vi "Register Tool Buttons Pressed.vi"(8 "error in (no error)":errorcluster, 11 "UI Controller in":refnum<class "UI Controller.lvclass">) -> (0 "error out":errorcluster, 3 "UI Controller out":refnum<class "UI Controller.lvclass">)   [LabVIEW 2020, in "UI Controller.lvlib" / "UI Controller.lvclass"]
uses:
  UI Controller.lvclass
  C:/Program Files/National Instruments/LabVIEW 2020/vi.lib/ActorFrameworkMVC/Abstract Controller/Abstract Controller/Abstract Controller.lvclass
  C:/Program Files/National Instruments/LabVIEW 2020/vi.lib/ActorFramework/Actor/Actor.lvclass
  Views/Tools View/Tools View Messages/Register Tool Buttons Pressed Msg/Register Tool Buttons Pressed Msg.lvclass
  C:/Program Files/National Instruments/LabVIEW 2020/vi.lib/ActorFramework/Message/Message.lvclass
  Models/Map Model/Map Model Messages/Concrete Tool Buttons Pressed Msg/Concrete Tool Buttons Pressed Msg.lvclass
  C:/Program Files/National Instruments/LabVIEW 2020/vi.lib/ActorFrameworkObserver/Data Message/Data Message.lvclass
  <vilib>/ActorFramework/Message Enqueuer/Message Enqueuer.lvclass/Message Enqueuer.ctl
  Views/Map View/Map View Messages/Concrete Tool Buttons Pressed Msg/Concrete Tool Buttons Pressed Msg.lvclass
  UI Controller Messages/Concrete Tool Buttons Pressed Msg/Concrete Tool Buttons Pressed Msg.lvclass
  <vilib>/ActorFramework/Actor/Actor.lvclass/Actor.ctl
  <vilib>/ActorFramework/Message Enqueuer/Init from Existing Queue.vi
  <vilib>/ActorFramework/Message Priority Queue/Priority Enqueue.vi
  <vilib>/ActorFramework/Message Enqueuer/Message Enqueuer.lvclass
  <vilib>/ActorFrameworkMVC/Abstract Controller/Abstract Controller/Abstract Controller.lvclass
  <vilib>/ActorFramework/Actor/Actor.lvclass
panel:
  # "NOTICE -- YOU MUST LEAVE THIS NOTICE IN PLACE.\n\nCopyright (c) 2017, LIANG LIU Shawn.Liu.cn@gmail.com\nAll rights reserved.\n\nRedistribution and use in source and binary forms, with or without modification, are permitted provided that the following conditions are met:\n-Redistributions of source code must retain the above copyright notice, this list of conditions and the following disclaimer.\n-Redistributions in binary form must reproduce the above copyright notice, this list of conditions and the following disclaimer in the documentation and/or other materials provided with the distribution.\n-Neither the name of the eLp nor the names of its contributors may be used to endorse or promote products derived from this software without specific prior written permission.\n\nTHIS SOFTWARE IS PROVIDED BY THE COPYRIGHT HOLDERS AND CONTRIBUTORS \"AS IS\" AND ANY EXPRESS OR IMPLIED WARRANTIES, INCLUDING, BUT NOT LIMITED TO, THE IMPLIED WARRANTIES OF MERCHANTABILITY AND FITNESS FOR A PARTICULAR PURPOSE ARE DISCLAIMED. IN NO EVENT SHALL THE COPYRIGHT HOLDER OR CONTRIBUTORS BE LIABLE FOR ANY DIRECT, INDIRECT, INCIDENTAL, SPECIAL, EXEMPLARY, OR CONSEQUENTIAL DAMAGES (INCLUDING, BUT NOT LIMITED TO, PROCUREMENT OF SUBSTITUTE GOODS OR SERVICES; LOSS OF USE, DATA, OR PROFITS; OR BUSINESS INTERRUPTION) HOWEVER CAUSED AND ON ANY THEORY OF LIABILITY, WHETHER IN CONTRACT, STRICT LIABILITY, OR TORT (INCLUDING NEGLIGENCE OR OTHERWISE) ARISING IN ANY WAY OUT OF THE USE OF THIS SOFTWARE, EVEN IF ADVISED OF THE POSSIBILITY OF SUCH DAMAGE."
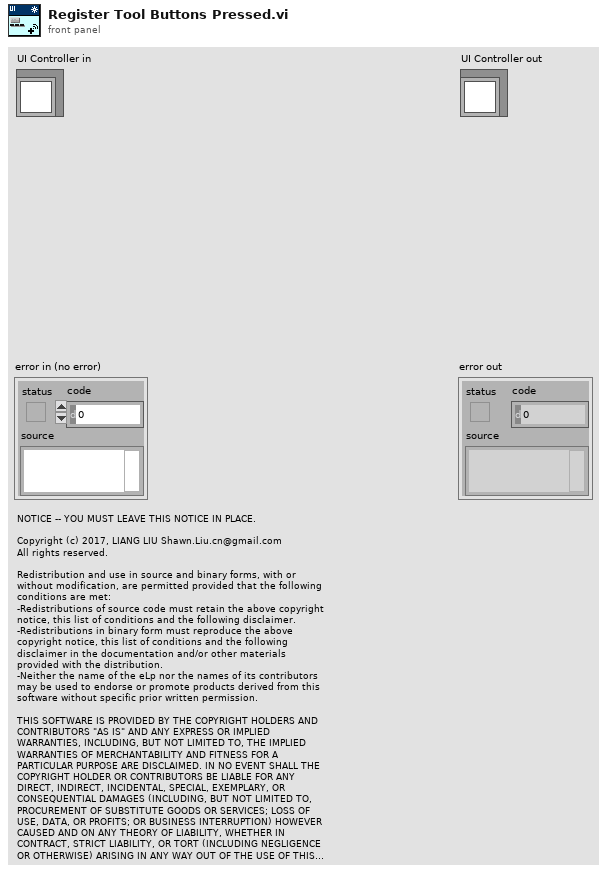
[diagram p1: front panel]
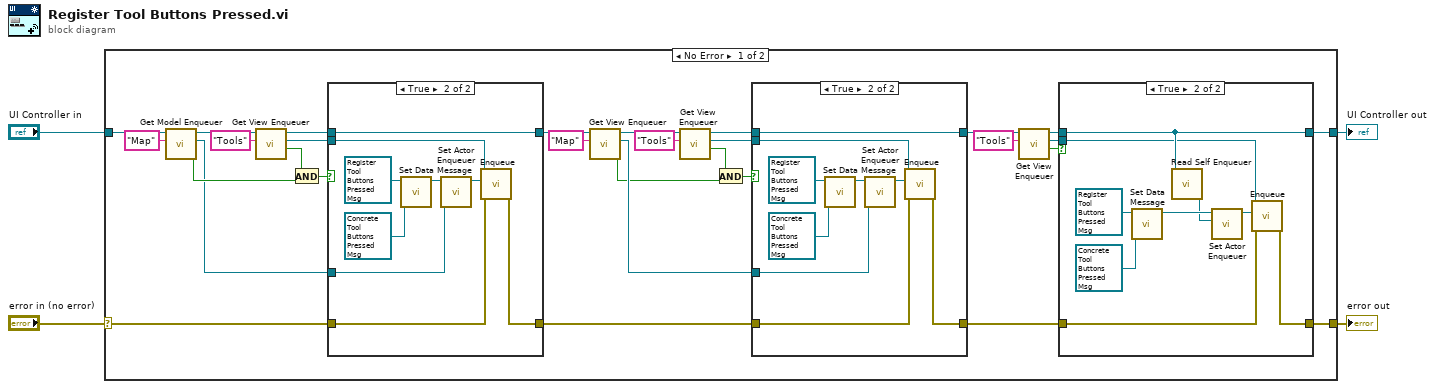
[diagram p0: block diagram]
diagram:
  n1 = case shown="No Error" "error in (no error)" {
    selector: "error in (no error)" -> [w33 w69]
    tunnel: "UI Controller in" -> [w34 w68]
    tunnel: [w6 w68] -> w2
    tunnel: [w5 w69] -> w1
    frame No Error {
      n2 = call <vilib>:"Get Model Enqueuer.vi"("Model Name"="Map", "Abstract Controller in"=w34) -> ("Found?"=w21:bool, "Model Enqueuer"=w20:refnum<class "Message Enqueuer.lvclass">, "Abstract Controller out"=w25:refnum<class "UI Controller.lvclass">)  [unwired: 6 in, 1 out]
      n3 = call <vilib>:"Get View Enqueuer.vi"("View Name"="Tools", "Abstract Controller in"=w25) -> ("Found?"=w22:bool, "View Enqueuer"=w27:refnum<class "Message Enqueuer.lvclass">, "Abstract Controller out"=w26:refnum<class "UI Controller.lvclass">)  [unwired: 6 in, 1 out]
      n4 = And(x=w22, y=w21) -> (x .and. y?=w23:bool)
      n5 = case shown="True" w23 {
        tunnel: w27 -> [_ w52]
        tunnel: w26 -> [w47 w53]
        tunnel: [w47 w53] -> w10
        tunnel: w33 -> [w46 w50]
        tunnel: [w46 w49] -> w9
        tunnel: w20 -> [_ w48]
        frame False {
        }
        frame True {
          n6 = call-dynamic "Set Data Message.vi"("Data Message"=refnum<class "Concrete Tool Buttons Pressed Msg.lvclass"> refnum ("Map Model.lvlib:Concrete Tool Buttons Pressed Msg.lvclass"), "Registration Message in"=refnum<class "Register Tool Buttons Pressed Msg.lvclass"> refnum ("Tools View.lvlib:Register Tool Buttons Pressed Msg.lvclass")) -> ("Registration Message out"=w55:refnum<class "Register Tool Buttons Pressed Msg.lvclass">)  [unwired: 9 in]
          n7 = call-dynamic "Set Actor Enqueuer.vi"("Actor Enqueuer"=w48, "Registration Message in"=w55) -> ("Registration Message out"=w51:refnum<class "Register Tool Buttons Pressed Msg.lvclass">)  [unwired: 9 in]
          n8 = call <vilib>:"Enqueue.vi"("error in (no error)"=w50, "Message"=w51, "Message Enqueuer in"=w52) -> ("error out"=w49:errorcluster)  [unwired: 7 in, 1 out]
        }
      }
      n9 = call <vilib>:"Get View Enqueuer.vi"("View Name"="Map" ("Model Name"), "Abstract Controller in"=w10) -> ("Found?"=w18:bool, "View Enqueuer"=w19:refnum<class "Message Enqueuer.lvclass">, "Abstract Controller out"=w14:refnum<class "UI Controller.lvclass">)  [unwired: 6 in, 1 out]
      n10 = call <vilib>:"Get View Enqueuer.vi"("View Name"="Tools", "Abstract Controller in"=w14) -> ("Found?"=w17:bool, "View Enqueuer"=w12:refnum<class "Message Enqueuer.lvclass">, "Abstract Controller out"=w13:refnum<class "UI Controller.lvclass">)  [unwired: 6 in, 1 out]
      n11 = And(x=w17, y=w18) -> (x .and. y?=w16:bool)
      n12 = case shown="True" w16 {
        tunnel: w12 -> [_ w41]
        tunnel: w13 -> [w36 w42]
        tunnel: [w36 w42] -> w8
        tunnel: w9 -> [w35 w39]
        tunnel: [w35 w38] -> w7
        tunnel: w19 -> [_ w37]
        frame False {
        }
        frame True {
          n13 = call-dynamic "Set Data Message.vi"("Data Message"=refnum<class "Concrete Tool Buttons Pressed Msg.lvclass"> refnum ("Map View.lvlib:Concrete Tool Buttons Pressed Msg.lvclass"), "Registration Message in"=refnum<class "Register Tool Buttons Pressed Msg.lvclass"> refnum ("Tools View.lvlib:Register Tool Buttons Pressed Msg.lvclass")) -> ("Registration Message out"=w44:refnum<class "Register Tool Buttons Pressed Msg.lvclass">)  [unwired: 9 in]
          n14 = call-dynamic "Set Actor Enqueuer.vi"("Actor Enqueuer"=w37, "Registration Message in"=w44) -> ("Registration Message out"=w40:refnum<class "Register Tool Buttons Pressed Msg.lvclass">)  [unwired: 9 in]
          n15 = call <vilib>:"Enqueue.vi"("error in (no error)"=w39, "Message"=w40, "Message Enqueuer in"=w41) -> ("error out"=w38:errorcluster)  [unwired: 7 in, 1 out]
        }
      }
      n16 = call <vilib>:"Get View Enqueuer.vi"("View Name"="Tools", "Abstract Controller in"=w8) -> ("Found?"=w31:bool, "View Enqueuer"=w30:refnum<class "Message Enqueuer.lvclass">, "Abstract Controller out"=w29:refnum<class "UI Controller.lvclass">)  [unwired: 6 in, 1 out]
      n17 = case shown="True" w31 {
        tunnel: w30 -> [_ w62]
        tunnel: w29 -> [w58 w63]
        tunnel: [w58 w63] -> w6
        tunnel: w7 -> [w57 w60]
        tunnel: [w57 w59] -> w5
        frame False {
        }
        frame True {
          n18 = call-dynamic "Set Data Message.vi"("Data Message"=refnum<class "Concrete Tool Buttons Pressed Msg.lvclass"> refnum ("UI Controller.lvlib:Concrete Tool Buttons Pressed Msg.lvclass"), "Registration Message in"=refnum<class "Register Tool Buttons Pressed Msg.lvclass"> refnum ("Tools View.lvlib:Register Tool Buttons Pressed Msg.lvclass")) -> ("Registration Message out"=w66:refnum<class "Register Tool Buttons Pressed Msg.lvclass">)  [unwired: 9 in]
          n19 = call <vilib>:"Read Self Enqueuer.vi"("Actor"=w63) -> ("Self Enqueuer"=w64:refnum<class "Message Enqueuer.lvclass">)  [unwired: 10 in]
          n20 = call-dynamic "Set Actor Enqueuer.vi"("Actor Enqueuer"=w64, "Registration Message in"=w66) -> ("Registration Message out"=w61:refnum<class "Register Tool Buttons Pressed Msg.lvclass">)  [unwired: 9 in]
          n21 = call <vilib>:"Enqueue.vi"("error in (no error)"=w60, "Message"=w61, "Message Enqueuer in"=w62) -> ("error out"=w59:errorcluster)  [unwired: 7 in, 1 out]
        }
      }
    }
    frame Error {
    }
  }
  "error out" <- w1
  "UI Controller out" <- w2
